vi "Send-priority-message.vi"(8 "error in (no error)":errorcluster, 9 "Receivers":T1[](array[typedef]), 10 "Message":refnum<class "Message.lvclass">, 11 "Client in":T2) -> (0 "error out":errorcluster, 3 "Client out":T2)   [LabVIEW 2013, in "SLMControl.lvlib" / "SC-Client.lvclass"]
doc: "Send a message to the specified list of receivers.\nThe message is added to the front of the server message queue and will be treated with priority.\nThe message needs to be created beforehand, either manually or through the 'Create-message' function and any specific contents need to be pre-configured. This function takes care of the sender and time information.\nThe receivers must be provided as an array. Each receiver entry can be composed in two ways: either '<module type>' to send to all active clients of the specified type, or '<module type><module ID>' to send to a specific client. Optionally the special client types 'All' or 'Server' can be used to send the message to all active clients (server excluded) or to the server, respectively."
uses:
  SC-Client.lvclass
  Object-reference.ctl
  SA-SLMAPI/Sources/Message.lvclass
  Supported-modules.ctl
  SC-Client.lvclass/SC-Client.ctl
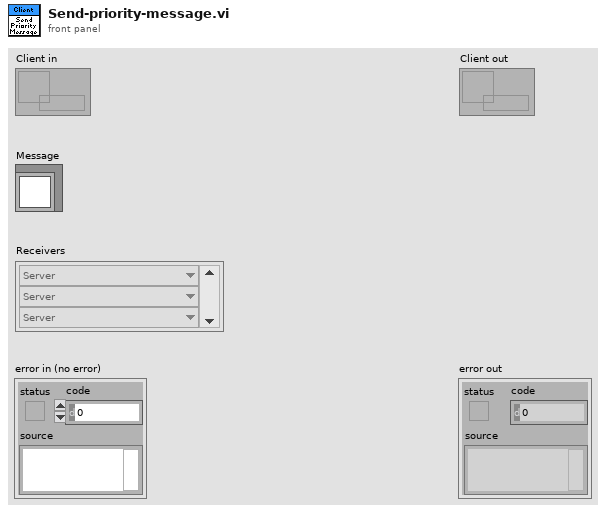
[diagram p1: front panel]
types:
  T1 = typedef "SLMControl.lvlib/SC-Client.lvclass/Supported-modules.ctl" = enum16{"Server", "All", "SLMControl", "PowderDeposition", "StrategyParser", "CameraVision", "MaterialCharacterization", "StatusMonitor", "SLMSimulation", "LaserCharacterization"}
  T2 = typedef "SLMControl.lvlib/SC-Client.lvclass/Object-reference.ctl" = refnum<data-value>
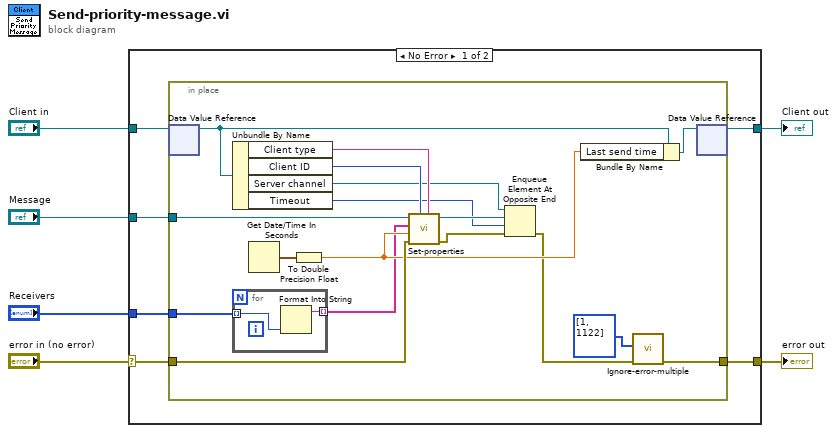
[diagram p0: block diagram]
diagram:
  n1 = case shown="No Error" "error in (no error)" {
    selector: "error in (no error)" -> [w8 w33]
    tunnel: [w7 w33] -> w5
    tunnel: [w9 w32] -> w3
    tunnel: "Client in" -> [w10 w32]
    tunnel: "Message" -> [w12 _]
    tunnel: "Receivers" -> [w11 _]
    frame No Error {
      n2 = in-place {
        in-place-border: w12 -> [w29]
        in-place-border: w11 -> [w14]
        in-place-border: w8 -> [w27]
        in-place-border: [w15] -> w7
        n3 = in-place-dvr #1(w10) -> (w20:refnum<class "SC-Client.lvclass">)  [unwired: 1 out]
        n4 = Unbundle By Name(w20) -> ("Client type"=w25:string, "Client ID"=w26:i32, "Server channel"=w21:refnum<queue>, "Timeout"=w22:i32)
        n5 = for {
          tunnel: w14 -> [w31] mode=indexing
          tunnel: [w30] -> w13 mode=indexing
          n6 = Format Into String(w31) -> (resulting string=w30:string)  [unwired: 3 in, 1 out]
        }
        n7 = Get Date/Time In Seconds() -> (seconds since 1Jan1904=w28:timestamp)
        n8 = To Double Precision Float(number=w28) -> (double precision float=w18:dbl)
        n9 = call-dynamic "Set-properties.vi"("Sender type"=w25, "Sender ID"=w26, "error in (no error)"=w27, "Send time"=w18, "Receivers"=w13, "Message in"=w29) -> ("error out"=w23:errorcluster, "Message out"=w24:refnum<class "Message.lvclass">)  [unwired: 4 in]
        n10 = Enqueue Element At Opposite End(queue=w21, element=w24, timeout in ms (-1)=w22, error in (no error)=w23) -> (error out=w16:errorcluster)  [unwired: 2 out]
        n11 = Bundle By Name(cluster=w20, "Last send time"=w18) -> (w19:refnum<class "SC-Client.lvclass">)
        n12 = call "Ignore-error-multiple.vi"("error in (no error)"=w16, "Errors to ignore (1)"=i32[] [1, 1122]) -> ("error out"=w15:errorcluster)  [unwired: 9 in]
        n13 = in-place-dvr #1(w19) -> (w9:T2)  [unwired: 1 out]
      }
    }
    frame Error {
    }
  }
  "error out" <- w5
  "Client out" <- w3
